vi "Count Strings.vi"(10 "regular expression":string="^s", 11 "Array - String":string[](array[string])) -> (3 "Count":i32)   [LabVIEW 2021]
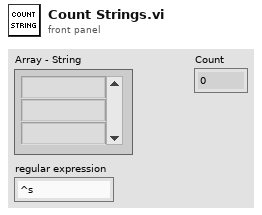
[diagram p1: front panel]
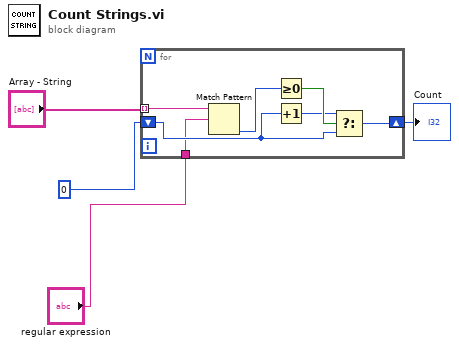
[diagram p0: block diagram]
diagram:
  n1 = for {
    tunnel: "Array - String" -> [w11] mode=indexing
    shift-right: [w6] -> w1
    shift-left: 0 -> [w7]
    tunnel: "regular expression" -> [w5]
    n2 = Match Pattern(string=w11, regular expression=w5) -> (offset past match=w10:i32)  [unwired: 1 in, 3 out]
    n3 = Greater Or Equal To 0?(x=w10) -> (x >= 0?=w9:bool)
    n4 = Increment(x=w7) -> (x+1=w8:i32)
    n5 = Select(t=w8, s=w9, f=w7) -> (s? t:f=w6:i32)
  }
  "Count" <- w1
